vi "ma_SML RT Zoom FFT.vi"   [LabVIEW 2020, in "NI_MAPro.lvlib"]
uses:
  NI_MAPro.lvlib
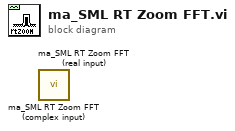
[diagram p0: block diagram]
diagram:
  n1 = call "ma_SML RT Zoom FFT (complex input).vi"() -> ()  [unwired: 7 in, 5 out]
  n2 = call "ma_SML RT Zoom FFT (real input).vi"() -> ()  [unwired: 7 in, 5 out]
